vi "Teamo72 Line Follow.vi"   [LabVIEW 2016]
uses:
  <vilib>/NXT/Subs/MotorOutput.ctl
  <vilib>/NXT/Block Support/NXT_InputPort.ctl
  <vilib>/NXT/Subs/LVHSConnector.ctl
  <vilib>/NXT/LegoClasses/BrickReference/BrickReference.lvclass
  <vilib>/NXT/Block Support/NXT_ButtonSelector.ctl
  <vilib>/NXT/Dual Mode Library/Motors/MotorOn.vi
  <vilib>/NXT/Dual Mode Library/Sensors/Light_On.vi
  <vilib>/NXT/Dual Mode Library/Waits/Wait_Num(msec).vi
  <vilib>/NXT/Dual Mode Library/Sensors/Touch_Pressed.vi
  <vilib>/NXT/NXTIO Xnodes/NXTIONodeSubVIs/LEGOMoveAllMotorsDistance.vi
  <vilib>/NXT/NXTIO Xnodes/NXTIONodeSubVIs/LEGOStopAllMotors.vi
  <vilib>/NXT/Dual Mode Library/Display/drawText.vi
  <vilib>/NXT/NXTIO Xnodes/NXTIOXNode/NXTIO.xnode
  <vilib>/NXT/Hardware/Plugins/Open Port/OpenPortAddress.ctl
  <vilib>/NXT/Dual Mode Library/Sensors/readNXTButton.vi
  <vilib>/NXT/Dual Mode Library/Motors/MotorBrake.vi
types:
  T1 = typedef "LVHSConnector.ctl" = refnum<class "BrickReference.lvclass">
  T2 = typedef "MotorOutput.ctl" = u8
  T3 = typedef "NXT_InputPort.ctl" = u32
  T4 = typedef "NXT_ButtonSelector.ctl" = u16
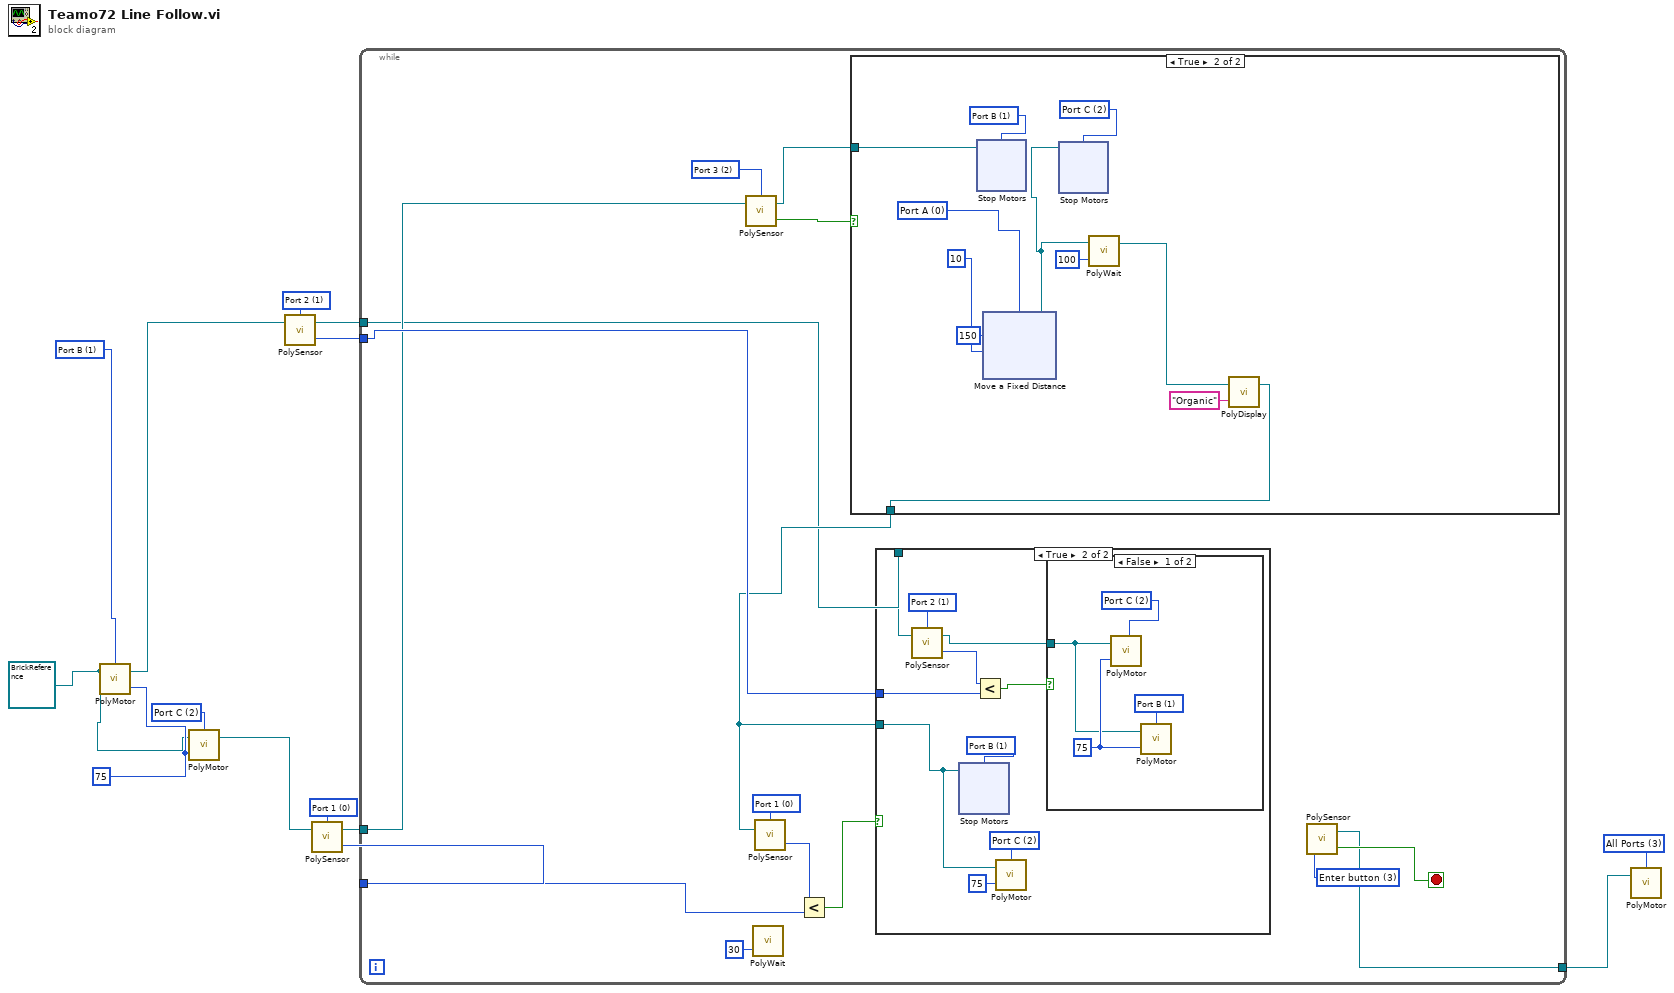
[diagram p0: block diagram]
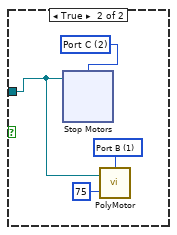
[diagram p4: hidden frame]
diagram:
  w5 = T1 refnum ("NXT/EV3")
  w8 = 75 ("Power (75)")
  w6 = T2 2 items=["Port A"=0, "Port B"=1, "Port C"=2, "Ports A & B"=4, "Ports A & C"=5, "Ports B & C"=6, "All Ports"=3] ("Output Port (All Ports)")
  w7 = T2 1 items=["Port A"=0, "Port B"=1, "Port C"=2, "Ports A & B"=4, "Ports A & C"=5, "Ports B & C"=6, "All Ports"=3] ("Output Port (All Ports)")
  w10 = T3 1 items=["Port 1", "Port 2", "Port 3", "Port 4"] ("Input Port (Port 3)")
  w12 = T2 3 items=["Port A"=0, "Port B"=1, "Port C"=2, "Ports A & B"=4, "Ports A & C"=5, "Ports B & C"=6, "All Ports"=3] ("Port (All Ports)")
  w13 = T3 0 items=["Port 1", "Port 2", "Port 3", "Port 4"] ("Input Port (Port 3)")
  n1 = call-poly <vilib>:"PolyMotor.vi"("Power (75)"=w8, "NXT/EV3"=w5, "Output Port (All Ports)"=w7) -> ("NXT/EV3"=w3:T1)  [unwired: 1 out]
  n2 = call-poly <vilib>:"PolyMotor.vi"("Power (75)"=w8, "NXT/EV3"=w5, "Output Port (All Ports)"=w6) -> ("NXT/EV3"=w4:T1)  [unwired: 1 out]
  n3 = call-poly <vilib>:"PolySensor.vi"("NXT/EV3"=w3, "Port (Port 3)"=w10) -> ("Scaled Value"=w9:i16, "NXT/EV3"=w2:T1)  [unwired: 1 out]
  n4 = call-poly <vilib>:"PolySensor.vi"("NXT/EV3"=w4, "Port (Port 3)"=w13) -> ("Scaled Value"=w14:i16, "NXT/EV3"=w1:T1)  [unwired: 1 out]
  n5 = while {
    tunnel: w14 -> [w22]
    tunnel: [w23] -> w11
    tunnel: w9 -> [w19]
    tunnel: w2 -> [w15]
    tunnel: w1 -> [w18]
    stop <- w24 stop-if-true
    w20 = T3 2 items=["Port 1", "Port 2", "Port 3", "Port 4"] ("Port (Port 1)")
    w25 = T4 3 items=["Enter button"=3, "Left button"=2, "Right button"=1] ("Button (Enter button)")
    w29 = T3 0 items=["Port 1", "Port 2", "Port 3", "Port 4"] ("Input Port (Port 3)")
    n6 = call-poly <vilib>:"PolySensor.vi"("NXT/EV3"=w18, "Port (Port 1)"=w20) -> ("Yes / No"=w21:bool, "NXT/EV3"=w17:T1)  [unwired: 1 in]
    n7 = call-poly <vilib>:"PolyWait.vi"("Time (100 msec)"=u32 30 ("Time (1 sec)")) -> ()  [unwired: 3 in, 1 out]
    n8 = case shown="True" w21 {
      tunnel: w17 -> [w30 w32]
      tunnel: [w30 w36] -> w16
      frame False {
      }
      frame True {
        w34 = T2 0 items=["Port A"=0, "Port B"=1, "Port C"=2, "Ports A & B"=4, "Ports A & C"=5, "Ports B & C"=6, "All Ports"=3] ("Output Port (All Ports)")
        w40 = T2 2 items=["Port A"=0, "Port B"=1, "Port C"=2, "Ports A & B"=4, "Ports A & C"=5, "Ports B & C"=6, "All Ports"=3] ("Output Port (All Ports)")
        w41 = T2 1 items=["Port A"=0, "Port B"=1, "Port C"=2, "Ports A & B"=4, "Ports A & C"=5, "Ports B & C"=6, "All Ports"=3] ("Output Port (All Ports)")
        n9 = xnode "Stop Motors"("Motors"=w41, "NXT/EV3"=w32) -> ()  [unwired: 1 out]
        n10 = xnode "Move a Fixed Distance"("Speed 1"=i8 10 ("Power/Speed 1"), "Distance 1"=150, "Motors"=w34) -> ("NXT/EV3"=w31:T1)  [unwired: 1 in]
        n11 = xnode "Stop Motors"("Motors"=w40, "NXT/EV3"=w31) -> ()  [unwired: 1 out]
        n12 = call-poly <vilib>:"PolyWait.vi"("Time (100 msec)"=u32 100, "NXT/EV3"=w31) -> ("NXT/EV3"=w37:T1)  [unwired: 2 in]
        n13 = call-poly <vilib>:"PolyDisplay.vi"("Text"="Organic", "NXT/EV3"=w37) -> ("NXT/EV3"=w36:T1)  [unwired: 2 in]
      }
    }
    n14 = call-poly <vilib>:"PolySensor.vi"("NXT/EV3"=w16, "Port (Port 3)"=w29) -> ("Scaled Value"=w27:i16)  [unwired: 2 out]
    n15 = Less?(x=w27, y=w22) -> (x < y?=w26:bool)
    n16 = case shown="True" w26 {
      tunnel: w19 -> [_ w66]
      tunnel: w15 -> [_ w64]
      tunnel: w16 -> [_ w62]
      frame False {
      }
      frame True {
        w68 = T3 1 items=["Port 1", "Port 2", "Port 3", "Port 4"] ("Input Port (Port 3)")
        w71 = T2 2 items=["Port A"=0, "Port B"=1, "Port C"=2, "Ports A & B"=4, "Ports A & C"=5, "Ports B & C"=6, "All Ports"=3] ("Output Port (All Ports)")
        w70 = T2 1 items=["Port A"=0, "Port B"=1, "Port C"=2, "Ports A & B"=4, "Ports A & C"=5, "Ports B & C"=6, "All Ports"=3] ("Output Port (All Ports)")
        n17 = call-poly <vilib>:"PolySensor.vi"("NXT/EV3"=w64, "Port (Port 3)"=w68) -> ("Scaled Value"=w67:i16, "NXT/EV3"=w63:T1)  [unwired: 1 out]
        n18 = xnode "Stop Motors"("Motors"=w70, "NXT/EV3"=w62) -> ()  [unwired: 1 out]
        n19 = Less?(x=w67, y=w66) -> (x < y?=w65:bool)
        n20 = call-poly <vilib>:"PolyMotor.vi"("Power (75)"=75, "NXT/EV3"=w62, "Output Port (All Ports)"=w71) -> ()  [unwired: 2 out]
        n21 = case shown="False" w65 {
          tunnel: w63 -> [w72 w76]
          frame False {
            w73 = 75 ("Power (75)")
            w75 = T2 1 items=["Port A"=0, "Port B"=1, "Port C"=2, "Ports A & B"=4, "Ports A & C"=5, "Ports B & C"=6, "All Ports"=3] ("Output Port (All Ports)")
            w74 = T2 2 items=["Port A"=0, "Port B"=1, "Port C"=2, "Ports A & B"=4, "Ports A & C"=5, "Ports B & C"=6, "All Ports"=3] ("Output Port (All Ports)")
            n22 = call-poly <vilib>:"PolyMotor.vi"("Power (75)"=w73, "NXT/EV3"=w72, "Output Port (All Ports)"=w74) -> ()  [unwired: 2 out]
            n23 = call-poly <vilib>:"PolyMotor.vi"("Power (75)"=w73, "NXT/EV3"=w72, "Output Port (All Ports)"=w75) -> ()  [unwired: 2 out]
          }
          frame True {
            w79 = T2 1 items=["Port A"=0, "Port B"=1, "Port C"=2, "Ports A & B"=4, "Ports A & C"=5, "Ports B & C"=6, "All Ports"=3] ("Output Port (All Ports)")
            w78 = T2 2 items=["Port A"=0, "Port B"=1, "Port C"=2, "Ports A & B"=4, "Ports A & C"=5, "Ports B & C"=6, "All Ports"=3] ("Output Port (All Ports)")
            n24 = xnode "Stop Motors"("Motors"=w78, "NXT/EV3"=w76) -> ()  [unwired: 1 out]
            n25 = call-poly <vilib>:"PolyMotor.vi"("Power (75)"=75, "NXT/EV3"=w76, "Output Port (All Ports)"=w79) -> ()  [unwired: 2 out]
          }
        }
      }
    }
    n26 = call-poly <vilib>:"PolySensor.vi"("Button (Enter button)"=w25) -> ("Yes/No"=w24:bool, "NXT/EV3"=w23:T1)  [unwired: 1 in, 1 out]
  }
  n27 = call-poly <vilib>:"PolyMotor.vi"("NXT/EV3"=w11, "Port (All Ports)"=w12) -> ()  [unwired: 3 out]
